vi "delete channel from SHM configuration.vi"(8 "error in":errorcluster, 10 "channel to delete":string, 11 "SHM configuration in":refnum<class "Shared Memory configuration.lvclass">) -> (0 "error out":errorcluster, 3 "SHM configuration out":refnum<class "Shared Memory configuration.lvclass">)   [LabVIEW 2013, in "Shared Memory configuration.lvclass"]
uses:
  module/configuration/Shared Memory configuration.lvclass
  module/configuration/Shared Memory configuration.lvclass/Shared Memory configuration.ctl
  <vilib>/NI/Tag Bus/tag/tag descriptor.lvclass/tag descriptor.ctl
  <vilib>/NI/Tag Bus/tag/read tag name.vi
  <vilib>/NI/Tag Bus/tag/tag descriptor.lvclass
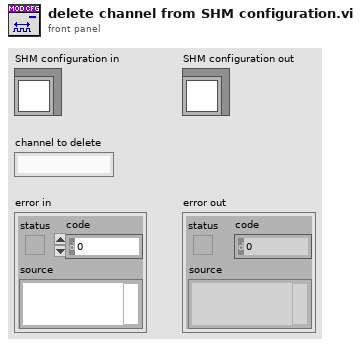
[diagram p1: front panel]
types:
  T1 = typedef "Shared Memory configuration.lvclass/Line.ctl" = cluster{"channel":refnum<class "TBM channel.lvclass">}
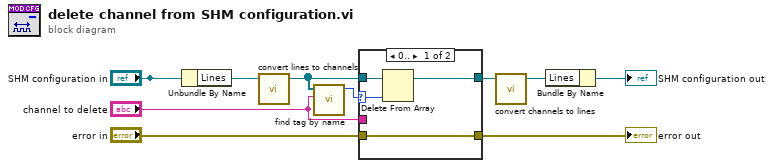
[diagram p0: block diagram]
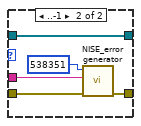
[diagram p2: hidden frame]
diagram:
  n1 = Unbundle By Name("SHM configuration in") -> ("Lines"=w5:T1[])
  n2 = call "convert lines to channels.vi"("Lines in"=w5) -> ("channels out"=w4:refnum<class "TBM channel.lvclass">[])  [unwired: 9 in, 1 out]
  n3 = call <vilib>:"find tag by name.vi"("name"="channel to delete", "tags in"=w4) -> ("index"=w8:i32)  [unwired: 9 in]
  n4 = case shown="0.." w8 {
    selector: w8 -> [w13 _]
    tunnel: [w12 w18] -> w3
    tunnel: w4 -> [w14 w18]
    tunnel: "error in" -> [w11 w17]
    tunnel: [w11 w16] -> w6
    tunnel: "channel to delete" -> [_ w15]
    frame 0.. {
      n5 = Delete From Array(array=w14, index=w13) -> (array with subset deleted=w12:refnum<class "TBM channel.lvclass">[])  [unwired: 1 in, 1 out]
    }
    frame ..-1 {
      n6 = call <vilib>:"NISE_error generator.vi"("error in"=w17, "append error message"=w15, "error code (0)"=538351) -> ("error out"=w16:errorcluster)  [unwired: 6 in]
    }
  }
  "error out" <- w6
  n7 = call "convert channels to lines.vi"("channels"=w3) -> ("Lines"=w2:T1[])  [unwired: 9 in, 1 out]
  n8 = Bundle By Name(cluster="SHM configuration in", "Lines"=w2) -> (→"SHM configuration out":refnum<class "Shared Memory configuration.lvclass">)
